vi "Read fpga res type.vi"(8 "error in (no error)":errorcluster, 11 "Fxp Channel in":refnum<class "FPGA Channel.lvclass">) -> (0 "error out":errorcluster, 2 "fpga res type":T1, 3 "Fxp Channel out":refnum<class "FPGA Channel.lvclass">)   [LabVIEW 2014, in "FPGA Channel.lvclass"]
uses:
  FPGA Channel.lvclass
  fpga resource supported data types.ctl
  FPGA Channel.lvclass/FPGA Channel.ctl
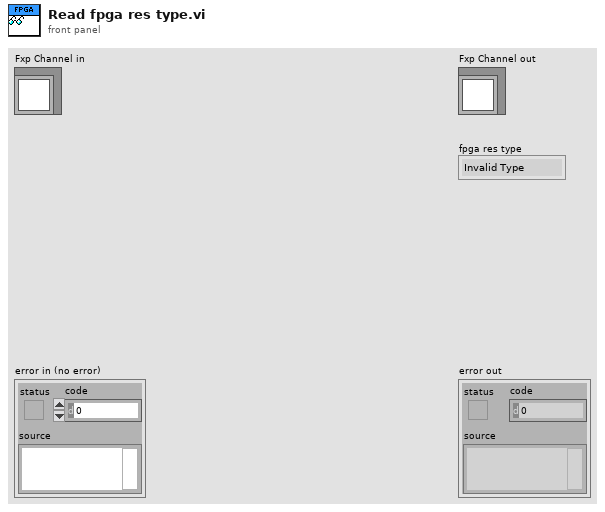
[diagram p1: front panel]
types:
  T1 = typedef "FPGA Channel.lvclass/fpga resource supported data types.ctl" = enum16{"Invalid Type", "Single", "I64", "I32", "I16", "I8", "U64", "U32", "U16", "U8", "Boolean", "FXP I,20,5", "FXP I,24,5", "FXP I,24,10", "Fifo 1023,I16"}
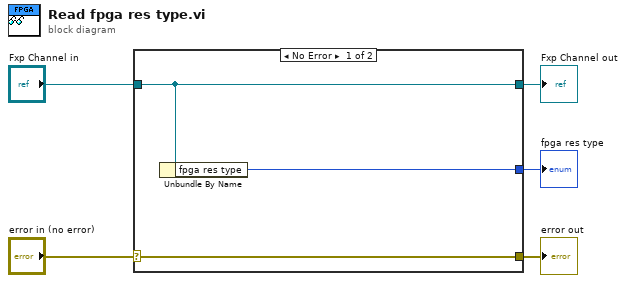
[diagram p0: block diagram]
diagram:
  n1 = case shown="No Error" "error in (no error)" {
    selector: "error in (no error)" -> [w8 w9]
    tunnel: [w8 w9] -> w4
    tunnel: [w7 w10] -> w2
    tunnel: "Fxp Channel in" -> [w7 w10]
    tunnel: [w6 _] -> w1
    frame No Error {
      n2 = Unbundle By Name(w7) -> ("fpga res type"=w6:T1)
    }
    frame Error {
    }
  }
  "error out" <- w4
  "Fxp Channel out" <- w2
  "fpga res type" <- w1
